vi "GetConfigurationString.vi"(8 "ErrorIn":errorcluster, 10 "Identification":string, 11 "ReferenceIn":refnum<class "AppConfigJSON.lvclass">) -> (0 "ErrorOut":errorcluster, 2 "String":string, 3 "ReferenceOut":refnum<class "AppConfigJSON.lvclass">)   [LabVIEW 2021, in "AppConfigJSON.lvclass"]
uses:
  AppConfigJSON.lvclass
  AppConfigJSON.lvclass/AppConfigJSON.ctl
  <vilib>/JDP Science/JSONtext/Config Files/Config File.lvclass
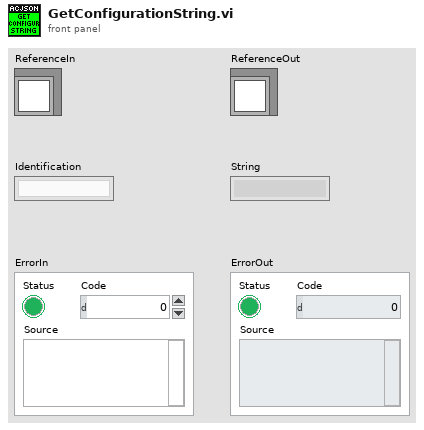
[diagram p1: front panel]
types:
  T1 = typedef "AppConfigJSON.lvclass/ObjectAttributes.ctl" = cluster{"Name":string, "ConfigFilePath":path, "Objects":T2[], "ApplicationBasePath":path, "ObjectName":string}
  T2 = typedef "IApplicationConfiguration.lvclass/ObjectDataDetails.ctl" = cluster{"ObjectName":string, "ObjectType":string, "Interfaces":T3[]}
  T3 = typedef "IApplicationConfiguration.lvclass/ObjectData.ctl" = cluster{"Label":string, "ObjectName":string, "Type":string}
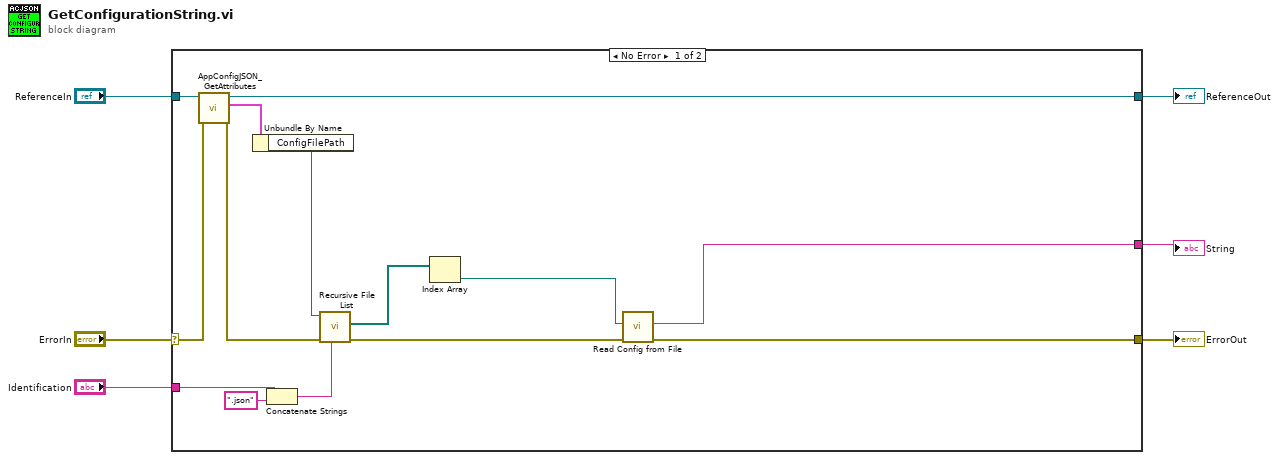
[diagram p0: block diagram]
diagram:
  n1 = case shown="No Error" "ErrorIn" {
    selector: "ErrorIn" -> [w18 w20]
    tunnel: [w17 w20] -> w5
    tunnel: [w14 w19] -> w3
    tunnel: "ReferenceIn" -> [w15 w19]
    tunnel: [w13 _] -> w2
    tunnel: "Identification" -> [w11 _]
    frame No Error {
      n2 = call "AppConfigJSON_GetAttributes.vi"("ErrorIn"=w18, "ReferenceIn"=w15) -> ("ErrorOut"=w17:errorcluster, "Data"=w16:T1, "ReferenceOut"=w14:refnum<class "AppConfigJSON.lvclass">)  [unwired: 6 in, 1 out]
      n3 = Unbundle By Name(w16) -> ("ConfigFilePath"=w12:path)
      n4 = Concatenate Strings(w11, ".json" ("string")) -> (w9:string)
      n5 = call <vilib>:"Recursive File List.vi"("pattern"=w9, "error in (no error)"=w17, "Folder Path"=w12) -> ("All Files in Dir"=w8:path[])  [unwired: 4 in, 4 out]
      n6 = Index Array(array=w8) -> (element=w7:path)  [unwired: 1 in]
      n7 = call <vilib>:"Read Config from File.vi"("error in (no error)"=w17, "config file path"=w7) -> ("<JSON>Config"=w13:string)  [unwired: 6 in, 3 out]
    }
    frame Error {
    }
  }
  "ErrorOut" <- w5
  "ReferenceOut" <- w3
  "String" <- w2
